vi "ODMR.vi"() -> ()   [LabVIEW 2025]
uses:
  <vilib>/Analysis/1siggen.llb/Ramp Pattern by Samples.vi
  <vilib>/DAQmx/write.llb/DAQmx Write (Analog 1D DBL NChan 1Samp).vi
  <vilib>/DAQmx/read.llb/DAQmx Read (Analog DBL 1Chan 1Samp).vi
  <vilib>/DAQmx/create/channels.llb/DAQmx Create Channel (AO-Voltage-Basic).vi
  <vilib>/DAQmx/miscellaneous.llb/DAQmx Fill In Error Info.vi
  <vilib>/DAQmx/create/channels.llb/DAQmx Create Channel (CI-Count Edges).vi
  <vilib>/DAQmx/configure/timing.llb/DAQmx Timing (Sample Clock).vi
  <vilib>/Analysis/NI_AALBase.lvlib
panel:
  in  "Y coordinate":i32
  in  "X coordinate":i32
  in  "Pixels":i32=128
  in  "Volts":dbl=10.0 format="%0.2f"
  out "XY Graph":cluster{"Y":dbl[], "Y":dbl[]}[](graph)
  in  "End frequency (Ghz)":dbl
  in  "Step size (Mhz)":dbl
  in  "start frequency (Ghz)":dbl
  in  "VISA resource name":refnum<visa-resource-name>
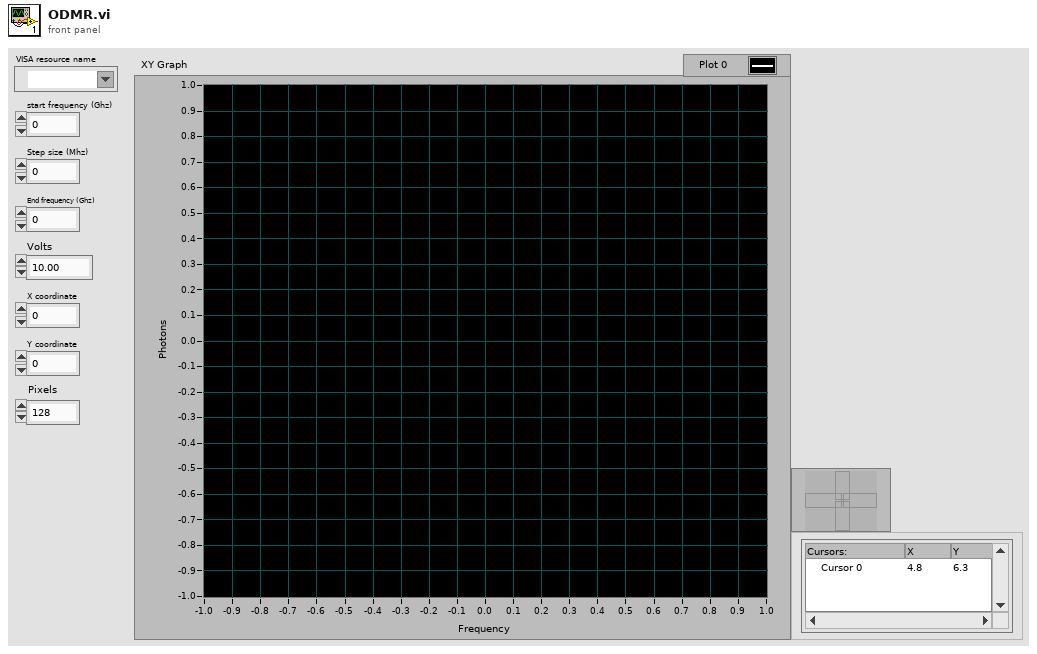
[diagram p1: front panel]
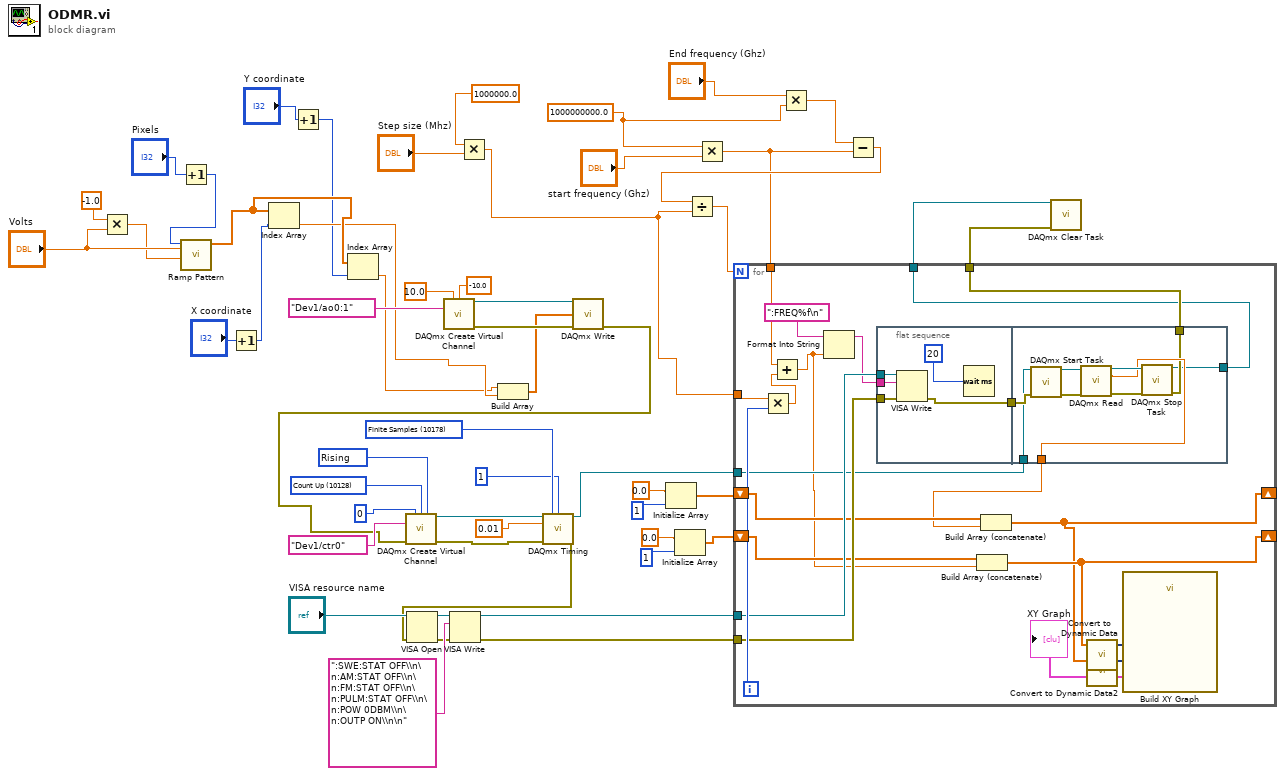
[diagram p0: block diagram]
diagram:
  w33 = 1000000000.0 ("x")
  w47 = 10178 items=["Finite Samples"=10178, "Continuous Samples"=10123, "Hardware Timed Single Point"=12522] ("sample mode")
  w49 = 10128 items=["Count Up"=10128, "Count Down"=10124, "Externally Controlled"=10326] ("count direction")
  w50 = 10280 items=["Rising"=10280, "Falling"=10171] ("edge")
  n1 = Multiply(x=-1.0, y="Volts") -> (x*y=w13:dbl)
  n2 = Increment(x="Pixels") -> (x+1=w11:i32)
  n3 = call-poly <vilib>:"Ramp Pattern.vi"("start"=w13, "end"="Volts", "samples"=w11) -> ("Ramp Pattern"=w7:dbl[])  [unwired: 7 in, 1 out]
  n4 = Increment(x="X coordinate") -> (x+1=w1:i32)
  n5 = Index Array(array=w7, index=w1) -> (element=w6:dbl)
  n6 = Increment(x="Y coordinate") -> (x+1=w3:i32)
  n7 = Index Array(array=w7, index=w3) -> (element=w5:dbl)
  n8 = call-poly <vilib>:"DAQmx Create Virtual Channel.vi"("maximum value"=10.0, "minimum value"=-10.0, "physical channels"=tag "Dev1/ao0:1") -> ("task out"=w54:refnum<k21>, "error out"=w41:errorcluster)  [unwired: 11 in]
  n9 = Multiply(x=1000000.0, y="Step size (Mhz)") -> (x*y=w28:dbl)
  n10 = Build Array(w5, w6) -> (w10:dbl[])
  n11 = call-poly <vilib>:"DAQmx Write.vi"("task/channels in"=w54, "data"=w10, "error in"=w41) -> ("error out"=w40:errorcluster)  [unwired: 10 in, 2 out]
  n12 = call-poly <vilib>:"DAQmx Create Virtual Channel.vi"("initial count"=u32 0, "count direction"=w49, "edge"=w50, "counter"=tag "Dev1/ctr0", "error in"=w40) -> ("task out"=w52:refnum<k21>, "error out"=w39:errorcluster)  [unwired: 9 in]
  n13 = call-poly <vilib>:"DAQmx Timing.vi"("task/channels in"=w52, "sample mode"=w47, "samples per channel"=1, "rate"=0.01, "error in"=w39) -> ("task out"=w24:refnum<k21>, "error out"=w38:errorcluster)  [unwired: 9 in]
  n14 = VISA Open(error in (no error)=w38, VISA resource name="VISA resource name") -> (VISA resource name=w43:refnum<visa-resource-name>, error out=w37:errorcluster)  [unwired: 3 in]
  n15 = VISA Write(VISA resource name=w43, write buffer=":SWE:STAT OFF\\n\n:AM:STAT OFF\\n\n:FM:STAT OFF\\n\n:PULM:STAT OFF\\n\n:POW 0DBM\\n\n:OUTP ON\\n\n", error in (no error)=w37) -> (VISA resource name out=w26:refnum<visa-resource-name>, error out=w25:errorcluster)  [unwired: 1 out]
  n16 = Initialize Array(0.0 ("element"), 1 ("dimension size")) -> (w23:dbl[])
  n17 = Initialize Array(0.0 ("element"), 1 ("dimension size")) -> (w18:dbl[])
  n18 = Multiply(x=w33, y="start frequency (Ghz)") -> (x*y=w27:dbl)
  n19 = Multiply(x="End frequency (Ghz)", y=w33) -> (x*y=w31:dbl)
  n20 = Subtract(x=w31, y=w27) -> (x-y=w30:dbl)
  n21 = Divide(x=w30, y=w28) -> (x/y=w29:dbl)
  n22 = for {
    N: w29 -> [_]
    tunnel: w28 -> [w73]
    tunnel: w27 -> [w72]
    tunnel: w26 -> [w70]
    tunnel: w25 -> [w68]
    tunnel: w24 -> [w66]
    shift-right: [w58] -> _
    shift-left: w23 -> [w65]
    shift-right: [w60] -> _
    shift-left: w18 -> [w64]
    tunnel: [w56] -> w17
    tunnel: [w55] -> w16
    i -> [w74]
    n23 = Multiply(x=w73, y=w74) -> (x*y=w75:dbl)
    n24 = Add(x=w72, y=w75) -> (x+y=w63:dbl)
    n25 = Format Into String(initial string=":FREQ%f\n", w63) -> (resulting string=w69:string)  [unwired: 2 in, 1 out]
    n26 = flat-sequence {
      tunnel: w70 -> [w80]
      tunnel: w69 -> [w79]
      tunnel: w68 -> [w78]
      tunnel: [w76] -> w67
      tunnel: w67 -> [w89]
      tunnel: w66 -> [w88]
      tunnel: [w83] -> w62
      tunnel: [w82] -> w56
      tunnel: [w81] -> w55
      frame #0 {
        n27 = VISA Write(VISA resource name=w80, write buffer=w79, error in (no error)=w78) -> (error out=w76:errorcluster)  [unwired: 2 out]
        n28 = Wait (ms)(milliseconds to wait=u32 20) -> ()  [unwired: 1 out]
      }
      frame #1 {
        n29 = call <vilib>:"DAQmx Start Task.vi"("task/channels in"=w88, "error in"=w89) -> ("task out"=w87:refnum<k21>, "error out"=w86:errorcluster)  [unwired: 12 in]
        n30 = call-poly <vilib>:"DAQmx Read.vi"("task/channels in"=w87, "error in"=w86) -> ("task out"=w84:refnum<k21>, "data"=w83:dbl, "error out"=w85:errorcluster)  [unwired: 11 in]
        n31 = call <vilib>:"DAQmx Stop Task.vi"("task/channels in"=w84, "error in"=w85) -> ("task out"=w81:refnum<k21>, "error out"=w82:errorcluster)  [unwired: 12 in]
      }
    }
    n32 = Build Array (concatenate)(w64, w63) -> (w60:dbl[])
    n33 = Build Array (concatenate)(w65, w62) -> (w58:dbl[])
    n34 = call "Convert to Dynamic Data"("Array"=w60) -> ("Dynamic Data Type"=w59:dynamicdata)  [unwired: 3 in]
    n35 = call "Convert to Dynamic Data2"("Array"=w58) -> ("Dynamic Data Type"=w57:dynamicdata)  [unwired: 3 in]
    n36 = call "Build XY Graph"("Y Input"=w57, "X Input"=w59) -> ("XY Graph"=→"XY Graph":cluster{"X":dbl[], "Y":dbl[]}[])  [unwired: 8 in, 1 out]
  }
  n37 = call <vilib>:"DAQmx Clear Task.vi"("task in"=w16, "error in"=w17) -> ()  [unwired: 13 in, 1 out]
